vi "opgave 3,1.vi"() -> ()   [LabVIEW 2015]
panel:
  out "Current Number":dbl
  in  "Number to Match":dbl=50.0 min=0.0 max=10000.0 step=1.0
  out "# of iterations":dbl
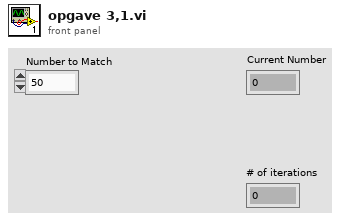
[diagram p1: front panel]
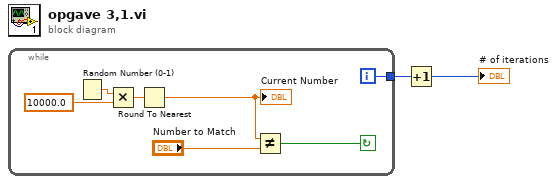
[diagram p0: block diagram]
diagram:
  n1 = while {
    tunnel: [w4] -> w2
    i -> [w4]
    stop <- w5 continue-if-true
    n2 = Random Number (0-1)() -> (number: 0 to 1=w6:dbl)
    n3 = Multiply(x=w6, y=10000.0) -> (x*y=w8:dbl)
    n4 = Round To Nearest(number=w8) -> (nearest integer value=w9:dbl)
    "Current Number" <- w9
    n5 = Not Equal?(x=w9, y="Number to Match") -> (x != y?=w5:bool)
  }
  n6 = Increment(x=w2) -> (x+1=→"# of iterations":i32)
